vi "Tunnel_Speed_Test.vi"() -> ()   [LabVIEW 2010]
panel:
  out "Waveform Graph":i32[](graph)
  in  "OGI Speed":dbl
  in  "stop":bool
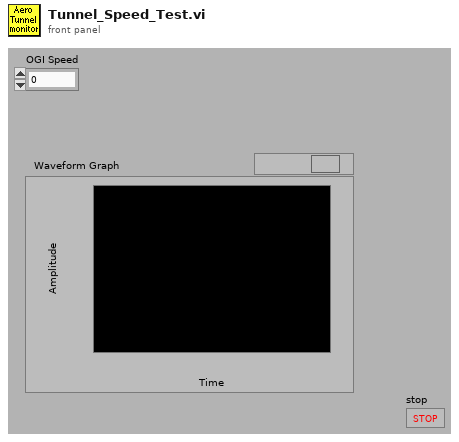
[diagram p1: front panel]
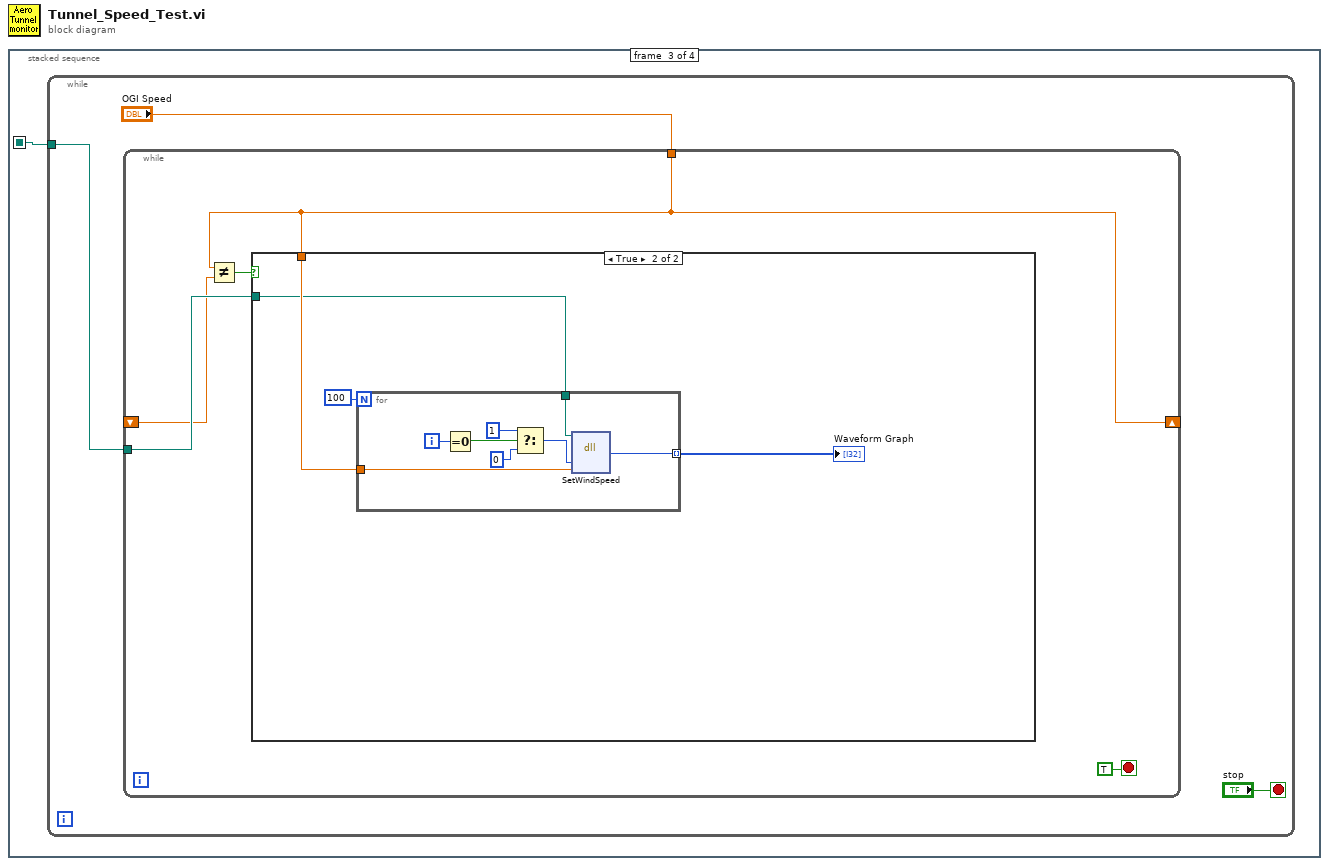
[diagram p0: block diagram]
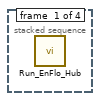
[diagram p2: hidden frame]
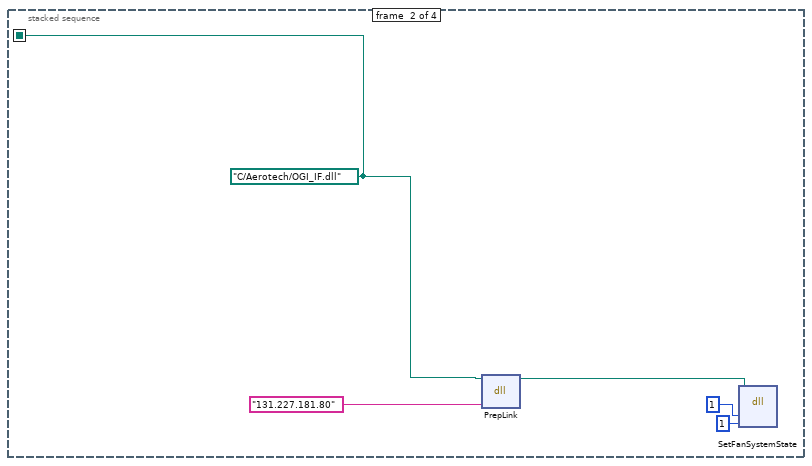
[diagram p3: hidden frame]
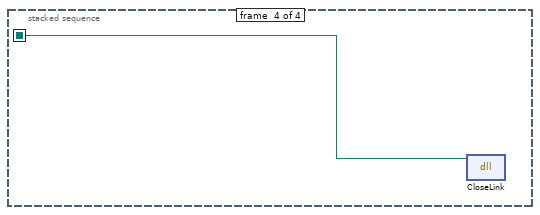
[diagram p5: hidden frame]
diagram:
  n1 = stacked-sequence {
    seq-local: [_ w4 _ _] -> [_ _ w6 w27]
    frame #0 {
      n2 = call "Run_EnFlo_Hub.vi"() -> ()  [unwired: 8 in]
    }
    frame #1 {
      w4 = path "C:/Aerotech/OGI_IF.dll" ("path in")
      n3 = dll-call lib="C:/Aerotech/Drivers/OGI_IF.dll" fn="PrepLink"(path in=w4, "IPAddress"="131.227.181.80") -> (path out=w2:path)  [unwired: 2 in, 3 out]
      n4 = dll-call lib="C:/Aerotech/Drivers/OGI_IF.dll" fn="SetFanSystemState"(path in=w2, "Enable"=1, "Fan ONOFF"=1) -> ()  [unwired: 3 in, 4 out]
    }
    frame #2 {
      n5 = while {
        tunnel: w6 -> [w9]
        stop <- "stop" stop-if-true
        n6 = while {
          tunnel: w9 -> [w14]
          tunnel: "OGI Speed" -> [w13]
          shift-right: [w13] -> _
          shift-left: _ -> [w12]
          stop <- TRUE stop-if-true
          n7 = Not Equal?(x=w13, y=w12) -> (x != y?=w10:bool)
          n8 = case shown="True" w10 {
            tunnel: w14 -> [_ w17]
            tunnel: w13 -> [_ w18]
            frame False {
            }
            frame True {
              n9 = for {
                N: 100 -> [_]
                tunnel: w18 -> [w26]
                tunnel: w17 -> [w25]
                tunnel: [w24] -> w15 mode=indexing
                i -> [w23]
                n10 = Equal To 0?(x=w23) -> (x = 0?=w22:bool)
                n11 = Select(t=1, s=w22, f=0 ("Enable")) -> (s? t:f=w19:i32)
                n12 = dll-call lib="C:/Aerotech/Drivers/OGI_IF.dll" fn="SetWindSpeed"(path in=w25, "Enable"=w19, "NewWindSpeed"=w26) -> ("Ack"=w24:i32)  [unwired: 4 in, 2 out]
              }
              "Waveform Graph" <- w15
            }
          }
        }
      }
    }
    frame #3 {
      n13 = dll-call lib="C:/Aerotech/Drivers/OGI_IF.dll" fn="CloseLink"(path in=w27) -> ()  [unwired: 2 in, 3 out]
    }
  }
